vi "SRV_Watchdog Build Commands Array.vi"(0 "System Config":T2={"SRV IP Address"="", "Video Stream Rate Period (ms)"=250, "Enable Diagnostic Log"=FALSE, "Watchdog 1 Config"={"Watchdog Name"="", "Watchdog Period (s)"=1.0, "Watchdog Command"={"I2C Address"=0, "Register"=0, "Value"=0, "Active"=FALSE}}, "Watchdog 2 Config"={"Watchdog Name"="", "Watchdog Period (s)"=1.0, "Watchdog Command"={"I2C Address"=0, "Register"=0, "Value"=0, "Active"=FALSE}}, "Sensor Window Filepath"=path ""} {"Watchdog 2 Config"."Watchdog Period (s)" format="%.3f"; "Watchdog 2 Config"."Watchdog Command"."Value" format="%02x"; "Watchdog 2 Config"."Watchdog Command"."Register" format="%02x"; "Watchdog 2 Config"."Watchdog Command"."I2C Address" format="%02x"; "Watchdog 1 Config"."Watchdog Period (s)" format="%.3f"; "Watchdog 1 Config"."Watchdog Command"."Value" format="%02x"; "Watchdog 1 Config"."Watchdog Command"."Register" format="%02x"; "Watchdog 1 Config"."Watchdog Command"."I2C Address" format="%02x"}, 7 "Update WD 1?":bool, 9 "Update WD 2?":bool, 11 "error in (no error)":errorcluster) -> (4 "System Config dup":T2={"SRV IP Address"="", "Video Stream Rate Period (ms)"=250, "Enable Diagnostic Log"=FALSE, "Watchdog 1 Config"={"Watchdog Name"="", "Watchdog Period (s)"=1.0, "Watchdog Command"={"I2C Address"=0, "Register"=0, "Value"=0, "Active"=FALSE}}, "Watchdog 2 Config"={"Watchdog Name"="", "Watchdog Period (s)"=1.0, "Watchdog Command"={"I2C Address"=0, "Register"=0, "Value"=0, "Active"=FALSE}}, "Sensor Window Filepath"=path ""} {"Watchdog 2 Config"."Watchdog Period (s)" format="%.3f"; "Watchdog 2 Config"."Watchdog Command"."Value" format="%02x"; "Watchdog 2 Config"."Watchdog Command"."Register" format="%02x"; "Watchdog 2 Config"."Watchdog Command"."I2C Address" format="%02x"; "Watchdog 1 Config"."Watchdog Period (s)" format="%.3f"; "Watchdog 1 Config"."Watchdog Command"."Value" format="%02x"; "Watchdog 1 Config"."Watchdog Command"."Register" format="%02x"; "Watchdog 1 Config"."Watchdog Command"."I2C Address" format="%02x"}, 8 "Watchdog Commands":T1[](array[typedef]) {"Value" format="%02x"; "Register" format="%02x"; "I2C Address" format="%02x"}, 15 "error out":errorcluster)   [LabVIEW 2014]
uses:
  SubVIs/SysConfig/SRV_System Config.ctl
  SRV_Watchdog Config Cluster.ctl
  Motors/Motors Config/SRV_Motor Control Command Config.ctl
panel:
  # "I2C Address"
  # "Register"
  # "Value"
  # "Active"
  # "I2C Address"
  # "Register"
  # "Value"
  # "Active"
  # "I2C Address"
  # "Register"
  # "Value"
  # "Active"
  # "I2C Address"
  # "Register"
  # "Value"
  # "Active"
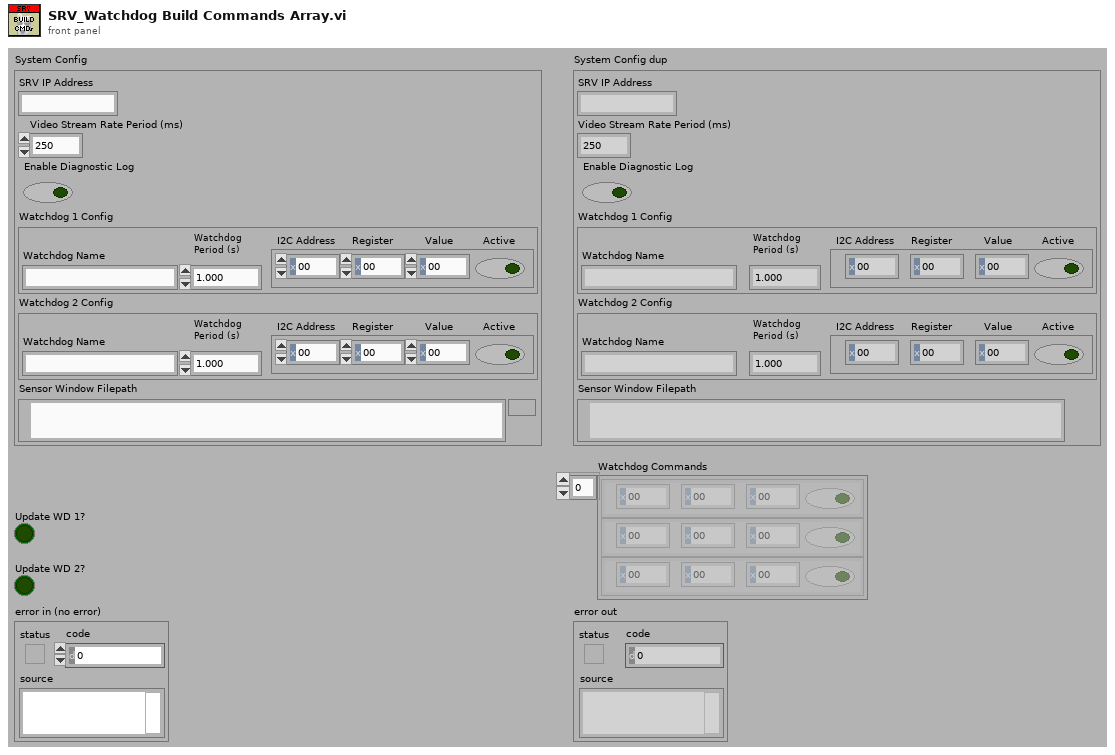
[diagram p1: front panel]
types:
  T1 = typedef "SRV_Motor Control Command Config.ctl" = cluster{"I2C Address":u8, "Register":u8, "Value":u8, "Active":bool}
  T2 = typedef "SRV_System Config.ctl" = cluster{"SRV IP Address":string, "Video Stream Rate Period (ms)":u32, "Enable Diagnostic Log":bool, "Watchdog 1 Config":T3, "Watchdog 2 Config":T3, "Sensor Window Filepath":path}
  T3 = typedef "SRV_Watchdog Config Cluster.ctl" = cluster{"Watchdog Name":string, "Watchdog Period (s)":dbl, "Watchdog Command":T1}
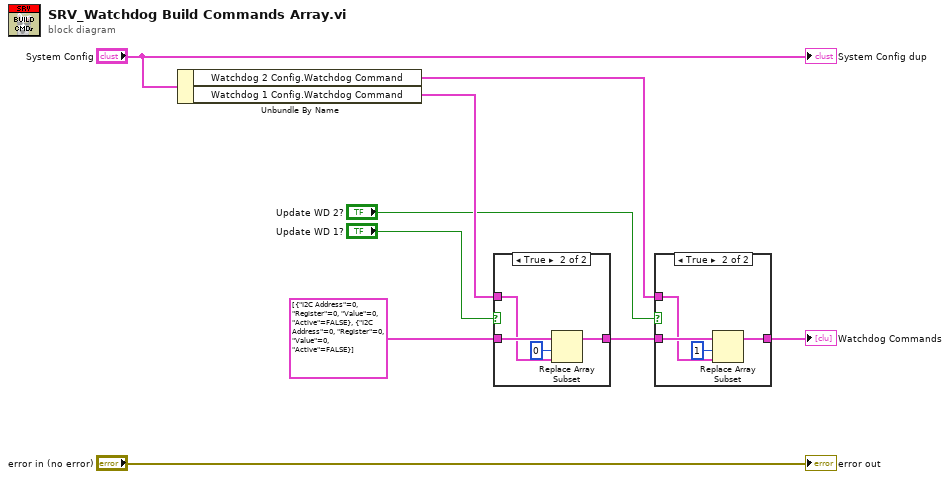
[diagram p0: block diagram]
diagram:
  n1 = Unbundle By Name("System Config") -> ("Watchdog 2 Config.Watchdog Command"=w2:T1, "Watchdog 1 Config.Watchdog Command"=w5:T1)
  n2 = case shown="True" "Update WD 1?" {
    tunnel: T1[] [{"I2C Address"=0, "Register"=0, "Value"=0, "Active"=FALSE}, {"I2C Address"=0, "Register"=0, "Value"=0, "Active"=FALSE}] ("Watchdog Commands") -> [w10 w14]
    tunnel: w5 -> [_ w11]
    tunnel: [w10 w13] -> w4
    frame False {
    }
    frame True {
      n3 = Replace Array Subset(array=w14, new element=w11, index=0) -> (w13:T1[])
    }
  }
  n4 = case shown="True" "Update WD 2?" {
    tunnel: w4 -> [w15 w19]
    tunnel: w2 -> [_ w16]
    tunnel: [w15 w18] -> w1
    frame False {
    }
    frame True {
      n5 = Replace Array Subset(array=w19, new element=w16, index=1) -> (w18:T1[])
    }
  }
  "Watchdog Commands" <- w1
  "error out" <- "error in (no error)"
  "System Config dup" <- "System Config"
